vi "Query Device Info.vi"(0 "PicoScope 3000a in":refnum<class "PicoScope 3000a.lvclass">, 11 "error in (no error)":errorcluster) -> (4 "PicoScope 3000a out":refnum<class "PicoScope 3000a.lvclass">, 15 "error out":errorcluster)   [LabVIEW 2018, in "PicoScope 3000a.lvlib" / "PicoScope 3000a.lvclass"]
uses:
  PicoScope 3000a.lvclass
  PicoScope 3000a.lvclass/PicoScope 3000a.ctl
  <instrlib>/PicoScope/PicoScope.lvlib
  ps3000a.dll
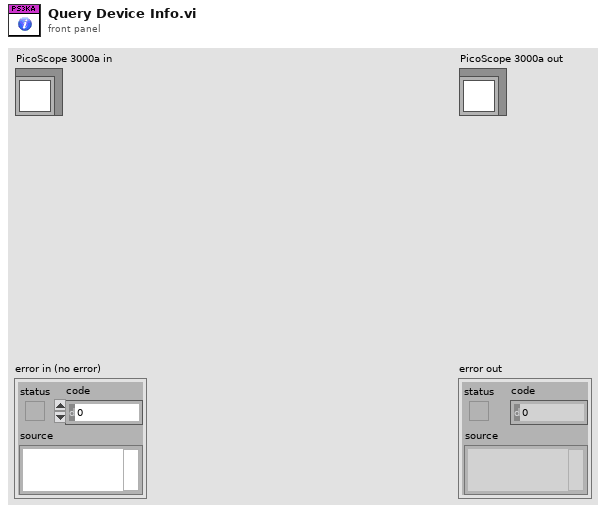
[diagram p1: front panel]
types:
  T1 = cluster{"Driver Version":string, "USB Version":string, "Hardware":string, "Variant":string, "Batch and Serial":string, "Cal Date":string, "Kernel Version":string, "Digital HW Version":string, "Analogue HW Version":string}
  T2 = cluster{"Driver Version":string, "USB Version":string, "Hardware":string, "Variant":string, "Batch and Serial":string, "Cal Date":string, "Kernel Version":string, "Digital HW Version":string, "Analogue HW Version":string, "MSO?":bool, "No. Channels":i16}
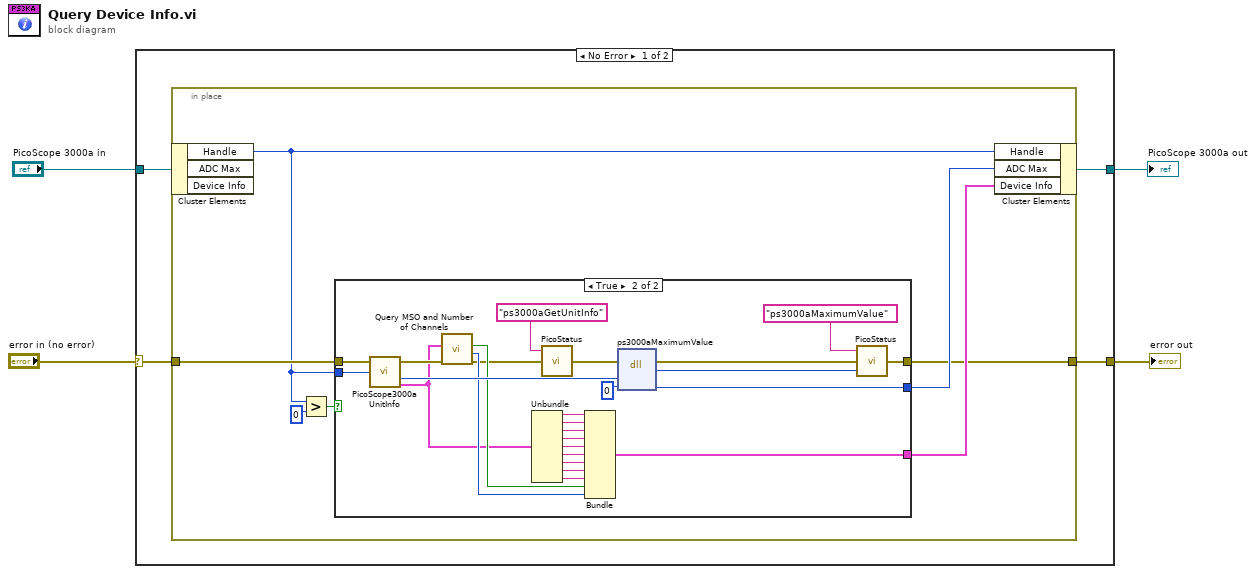
[diagram p0: block diagram]
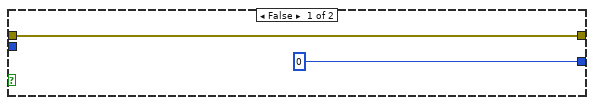
[diagram p2: hidden frame]
diagram:
  n1 = case shown="No Error" "error in (no error)" {
    selector: "error in (no error)" -> [w8 w45]
    tunnel: [w6 w45] -> w3
    tunnel: [w5 w44] -> w1
    tunnel: "PicoScope 3000a in" -> [w7 w44]
    frame No Error {
      n2 = in-place {
        in-place-border: w8 -> [w13]
        in-place-border: [w10] -> w6
        n3 = in-place-cluster #1(w7) -> ("Handle"=w9:i16)  [unwired: 2 out]
        n4 = Greater?(x=w9, y=i16 0) -> (0:w14:bool)
        n5 = case shown="True" w14 {
          tunnel: w9 -> [_ w43]
          tunnel: w13 -> [w17 w42]
          tunnel: [_ w25] -> w11
          tunnel: [i16 0 ("value") w24] -> w12
          tunnel: [w17 w23] -> w10
          frame False {
          }
          frame True {
            n6 = call <instrlib>:"PicoScope3000aUnitInfo.vi"("handle in"=w43, "error in (no error)"=w42) -> ("Unit Info"=w18:T1, "handle out"=w38:i16, "error out"=w20:errorcluster)  [unwired: 1 in]
            n7 = call "Query MSO and Number of Channels.vi"("error in (no error)"=w20, "Unit Info"=w18) -> ("error out"=w19:errorcluster, "No. Channels"=w21:i16, "MSO?"=w22:bool)  [unwired: 7 in]
            n8 = Unbundle(w18) -> ("Driver Version"=w34:string, "USB Version"=w33:string, "Hardware"=w32:string, "Variant"=w31:string, "Batch and Serial"=w30:string, "Cal Date"=w29:string, "Kernel Version"=w28:string, "Digital HW Version"=w27:string, "Analogue HW Version"=w26:string)
            n9 = call <instrlib>:"PicoStatus.vi"("error in"=w19, "source"="ps3000aGetUnitInfo") -> ("error out"=w36:errorcluster)  [unwired: 1 in]
            n10 = Bundle("Driver Version"=w34, "USB Version"=w33, "Hardware"=w32, "Variant"=w31, "Batch and Serial"=w30, "Cal Date"=w29, "Kernel Version"=w28, "Digital HW Version"=w27, "Analogue HW Version"=w26, "MSO?"=w22, "No. Channels"=w21) -> (w25:T2)  [unwired: 1 in]
            n11 = dll-call lib="ps3000a.dll" fn="ps3000aMaximumValue"(error in=w36, "handle"=w38, "value"=i16 0) -> (error out=w40:errorcluster, "PICO_STATUS"=w39:u32, "value"=w24:i16)  [unwired: 3 in, 1 out]
            n12 = call <instrlib>:"PicoStatus.vi"("PICO STATUS"=w39, "error in"=w40, "source"="ps3000aMaximumValue") -> ("error out"=w23:errorcluster)
          }
        }
        n13 = in-place-cluster #1("Handle"=w9, "ADC Max"=w12, "Device Info"=w11) -> (w5:refnum<class "PicoScope 3000a.lvclass">)
      }
    }
    frame Error {
    }
  }
  "error out" <- w3
  "PicoScope 3000a out" <- w1
